vi "Persist Entity.vi"(8 "error in (no error)":errorcluster, 10 "Conditum:Entity":refnum<class "Entity.lvclass">, 11 "Database in":refnum<class "Database Platform.lvclass">) -> (0 "error out":errorcluster, 3 "Database out":refnum<class "Database Platform.lvclass">)   [LabVIEW 2020, in "Conditum.lvlib" / "Database Platform.lvclass"]
uses:
  Database Platform.lvclass
  Entity/Entity.lvclass
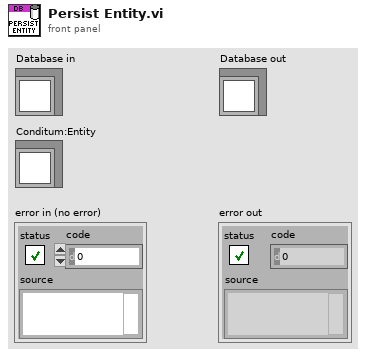
[diagram p1: front panel]
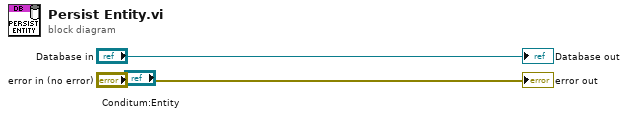
[diagram p0: block diagram]
diagram:
  "error out" <- "error in (no error)"
  "Database out" <- "Database in"
